vi "Ring Controls - Type Defs.vi"(6 "Numeric Constants":T1=3.141593 format="%#.6f" items=["NegativeInfinity"=-inf, "Pi"=3.141593, "NaturalLogarithmBase"=2.718282, "MolarGasConstant"=8.314472, "SpeedOfLightInVacuum "=299792458.0, "RydbergConstant"=10973731.568527, "NotANumber"=nan, "PostitiveInfinity"=inf], 7 "Enum":T6=enum."Three", 8 "Text & Picture":T3=9223372036854775807 items=["Home Sweet Home!"=9223372036854775807, "Zero In Chinese"=0, "Another Piece Of The Puzzle"=9000000006854770000, "Hmmm ????"=5729325037854735917, "The Connector Pane"=7213312035854725405, "Look At The Fish"=2513872035554745107, "Its A Turtle!"=1722372036854595802], 9 "Pict Ring Control":T2=2, 10 "Text Ring":T4=4 items=["Text Value 0", "Text Value 1", "Text Value 2", "Text Value 3", "Text Value 5", "Text Value 6"], 11 "Menu Ring":T5=33 items=["Menu Option 11"=11, "Menu Option 45"=45, "Menu Option 33"=33, "Menu Option 75"=75, "Menu Option 125"=125]) -> ()   [LabVIEW 2012]
uses:
  EnumTypeDefControl.ctl
  MenuRingTypeDefControl.ctl
  TextRingTypeDefControl.ctl
  Text&PictTypeDefControl.ctl
  PictRingTypeDefControl.ctl
  NumericConstantsControl.ctl
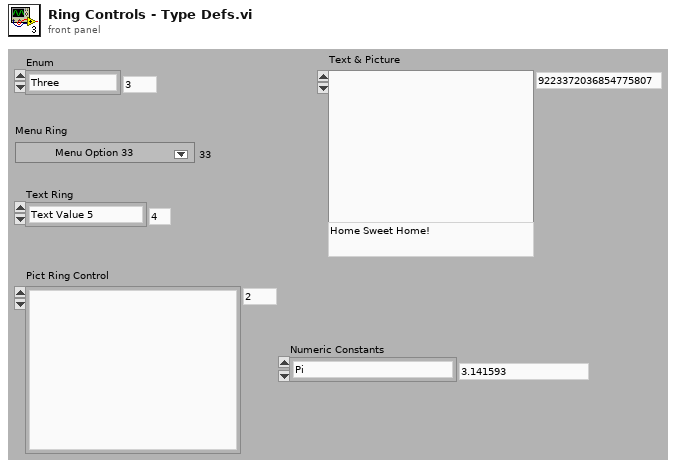
[diagram p1: front panel]
types:
  T1 = typedef "NumericConstantsControl.ctl" = dbl
  T2 = typedef "PictRingTypeDefControl.ctl" = u16
  T3 = typedef "Text&PictTypeDefControl.ctl" = i64
  T4 = typedef "TextRingTypeDefControl.ctl" = u16
  T5 = typedef "MenuRingTypeDefControl.ctl" = u32
  T6 = typedef "EnumTypeDefControl.ctl" = enum8{"Zero", "One", "Two", "Three", "Four", "Five"}
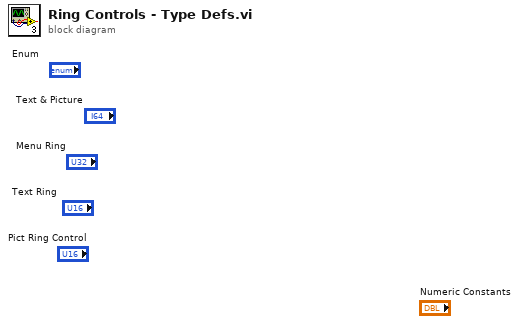
[diagram p0: block diagram]
diagram:
